vi "DMSO_EC_main_glass_cell_BM.vi"(0 "Constants":T5={"step to ml"=1920.0, "BoardNum"=1, "PosA BitNum"=6, "PosB BitNum"=5, "Heat Pulse Delay (ms)"=0.0, "Heating Iterations"=8, "N rinses"=2, "Dissolution Time (s)"=120, "SpargeBit"=0, "Extra Milli-Q (ml)"=2.0, "Valco Port Number"=6, "BitNum (Thermocouple)"=0, "Total Vol. (mL)"=12.0, "N syringe rinses"=2, "NaOH Vol (ml)"=2.0, "FanBit"=0}, 1 "Reduction Countdown Timer Refnum":refnum<vi>, 2 "Metadata":T1={"Local save location:"="C:\\Users\\bcamc\\OneDrive\\Desktop\\LabVIEW\\Test_metadata", "Cruise ID"="LaPerouse", "Sampling Timestamp"="2023-07-19 15:23:13", "Elution Timestamp"="2023-07-19 15:29:12", "GPS_Latitude"=-999.0, "GPS_Longitude"=-999.0, "DMS_std_conc"=0.0, "DMSP_std_conc"=0.0, "DMSO_std_conc"=0.0, "Std_index"=0.0, "Initial Trap Temp (oC)"=174.0, "Max Trap Temp (oC)"=174.0, "Final Trap Temp (oC)"=0.0, "Flow Rate (mL/min)"=0.0, "Comment"="", "GPS_Minute"=-999.0, "GPS_Day"=-999.0, "GPS_jd"=-999.0, "GPS_Hour"=-999.0, "GPS_Second"=-999.0, "GPS Baud"=4800.0, "COM Port (GPS)"="COM10", "Use GPS?"=FALSE, "Format Date"="%d-%d-%d"} {"GPS_Latitude" format="%_4g"; "GPS_Longitude" format="%_4g"; "GPS_jd" format="%_5g"; "Std_index" format="%.2g"; "DMSO_std_conc" format="%.2f"; "DMSP_std_conc" format="%.2f"; "DMS_std_conc" format="%.2f"}, 3 "Reduction Progress Bar Refnum":refnum<vi>, 4 "Sparging Countdown Timer Refnum":refnum<vi>, 5 "Sample Params":T4={"DMS Sparge Time (min)"=7.0, "Elution Time (min)"=1.5, "COM port (16 Pos. Valve)"="COM10", "Trap Heating Time (ms)"=675.0, "COM Port (DC Power)"="COM11", "COM Port (Runze)"="COM12", "sample volume"=10.0, "DMSO red. Sparge Time  (min)"=32.0, "DMSO Red. Duration (min)"=30.0, "Bypass sample handling (debugging)"=FALSE, "Reverse Reduction?"=FALSE, "Voltage (V)"="4.0", "DMSP Hydrolysis Time (min)"=13.0}, 6 "Sparging Progress Bar Refnum":refnum<vi>, 9 "Pump Parameters":T6={"Speed 1"="100", "Speed 2"="250", "Speed 3"="450", "Speed 4"="250", "UW/Sample"="5", "Sparge"="2", "Std"="4", "Waste"="15", "Air"="14", "Milli-Q"="1", "H2SO4"="6", "NaOH"="3", "Catalyst"="7", "Cell (H+ side)"="8", "Cell (sample side)"="9", "NaCl"="11"}, 10 "Elution Countdown Timer Refnum":refnum<vi>, 11 "Analysis Type":T3(ring)=enum."DMSO Only", 12 "Current Analyte Refnum":refnum<vi>, 14 "Temp Refnum":refnum<vi>, 15 "Elution Progress Bar Refnum":refnum<vi>) -> ()   [LabVIEW 2021]
uses:
  SubVIs/DMS-related/Sparge_stop.vi
  SubVIs/DMSO-related/Reduction_stop.vi
  SubVIs/DMS-related/Elution_stop.vi
  SubVIs/Refnum_control_global_BM.vi
  SubVIs/Plot_trap_heating_global_BM.vi
  SubVIs/DMSO-related/Temp_global_BM.vi
panel:
  out "Current Analyte":string
  in  "Mode Selection":T2(ring)
  out "Elution Progress Bar":u8(slide)=100 scale=0.0..100.0
  out "Sparging":bool
  out "Reduction Progress Bar":u8(slide)=100 scale=0.0..100.0
  out "Reduction Countdown (min)":dbl=-0.00026041666666666666 format="%.2g"
  out "Elution Countdown (min)":dbl=-0.0013020833333333333 format="%.2f"
  out "Error out":errorcluster
  out "Temp (oC)":i32=174
  in  "Error in":errorcluster
  out "Heating":bool
  out "Drying Flow":bool
  out "Sparge Countdown (min)":dbl=-0.00078125 format="%.2g"
  out "Sparging Progress Bar":u8(slide)=100 scale=0.0..100.0
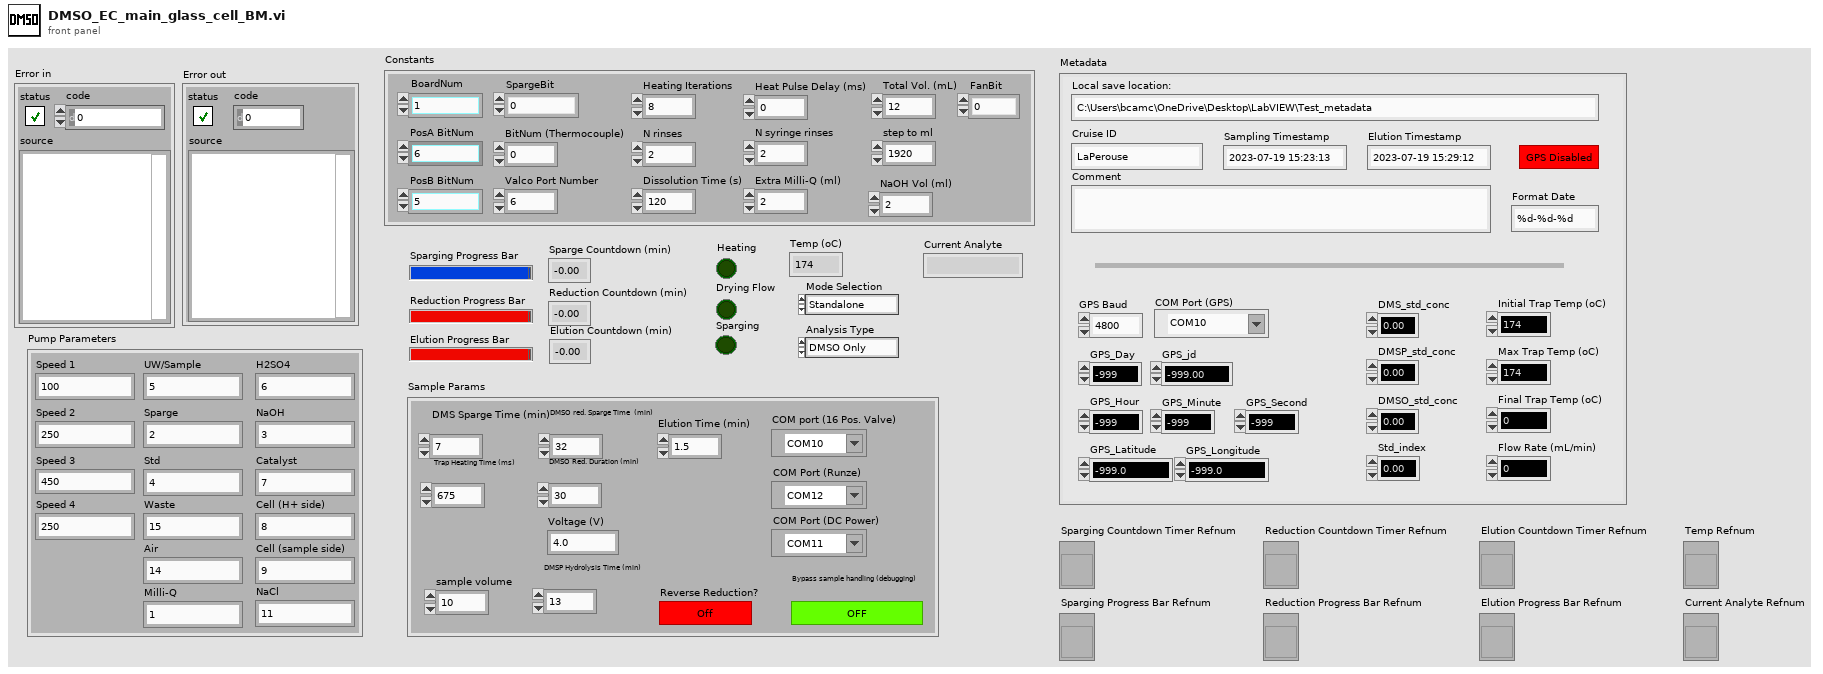
[diagram p1: front panel]
types:
  T1 = cluster{"Local save location:":string, "Cruise ID":string, "Sampling Timestamp":string, "Elution Timestamp":string, "GPS_Latitude":dbl, "GPS_Longitude":dbl, "DMS_std_conc":dbl, "DMSP_std_conc":dbl, "DMSO_std_conc":dbl, "Std_index":dbl, "Initial Trap Temp (oC)":dbl, "Max Trap Temp (oC)":dbl, "Final Trap Temp (oC)":dbl, "Flow Rate (mL/min)":dbl, "Comment":string, "GPS_Minute":dbl, "GPS_Day":dbl, "GPS_jd":dbl, "GPS_Hour":dbl, "GPS_Second":dbl, "GPS Baud":dbl, "COM Port (GPS)":refnum<visa-resource-name>, "Use GPS?":bool, "Format Date":string}
  T2 = enum16{"Standalone", "Standard Curve", "Point Std", "Analysis"}
  T3 = enum16{"DMS Only", "DMS/O", "DMS/P", "DMS/O/P", "DMSO Only"}
  T4 = cluster{"DMS Sparge Time (min)":dbl, "Elution Time (min)":dbl, "COM port (16 Pos. Valve)":refnum<visa-resource-name>, "Trap Heating Time (ms)":dbl, "COM Port (DC Power)":refnum<visa-resource-name>, "COM Port (Runze)":refnum<visa-resource-name>, "sample volume":dbl, "DMSO red. Sparge Time  (min)":dbl, "DMSO Red. Duration (min)":dbl, "Bypass sample handling (debugging)":bool, "Reverse Reduction?":bool, "Voltage (V)":string, "DMSP Hydrolysis Time (min)":dbl}
  T5 = cluster{"step to ml":dbl, "BoardNum":u32, "PosA BitNum":u32, "PosB BitNum":u32, "Heat Pulse Delay (ms)":dbl, "Heating Iterations":i32, "N rinses":i32, "Dissolution Time (s)":u32, "SpargeBit":u32, "Extra Milli-Q (ml)":dbl, "Valco Port Number":i32, "BitNum (Thermocouple)":u32, "Total Vol. (mL)":dbl, "N syringe rinses":i32, "NaOH Vol (ml)":dbl, "FanBit":u32}
  T6 = cluster{"Speed 1":string, "Speed 2":string, "Speed 3":string, "Speed 4":string, "UW/Sample":string, "Sparge":string, "Std":string, "Waste":string, "Air":string, "Milli-Q":string, "H2SO4":string, "NaOH":string, "Catalyst":string, "Cell (H+ side)":string, "Cell (sample side)":string, "NaCl":string}
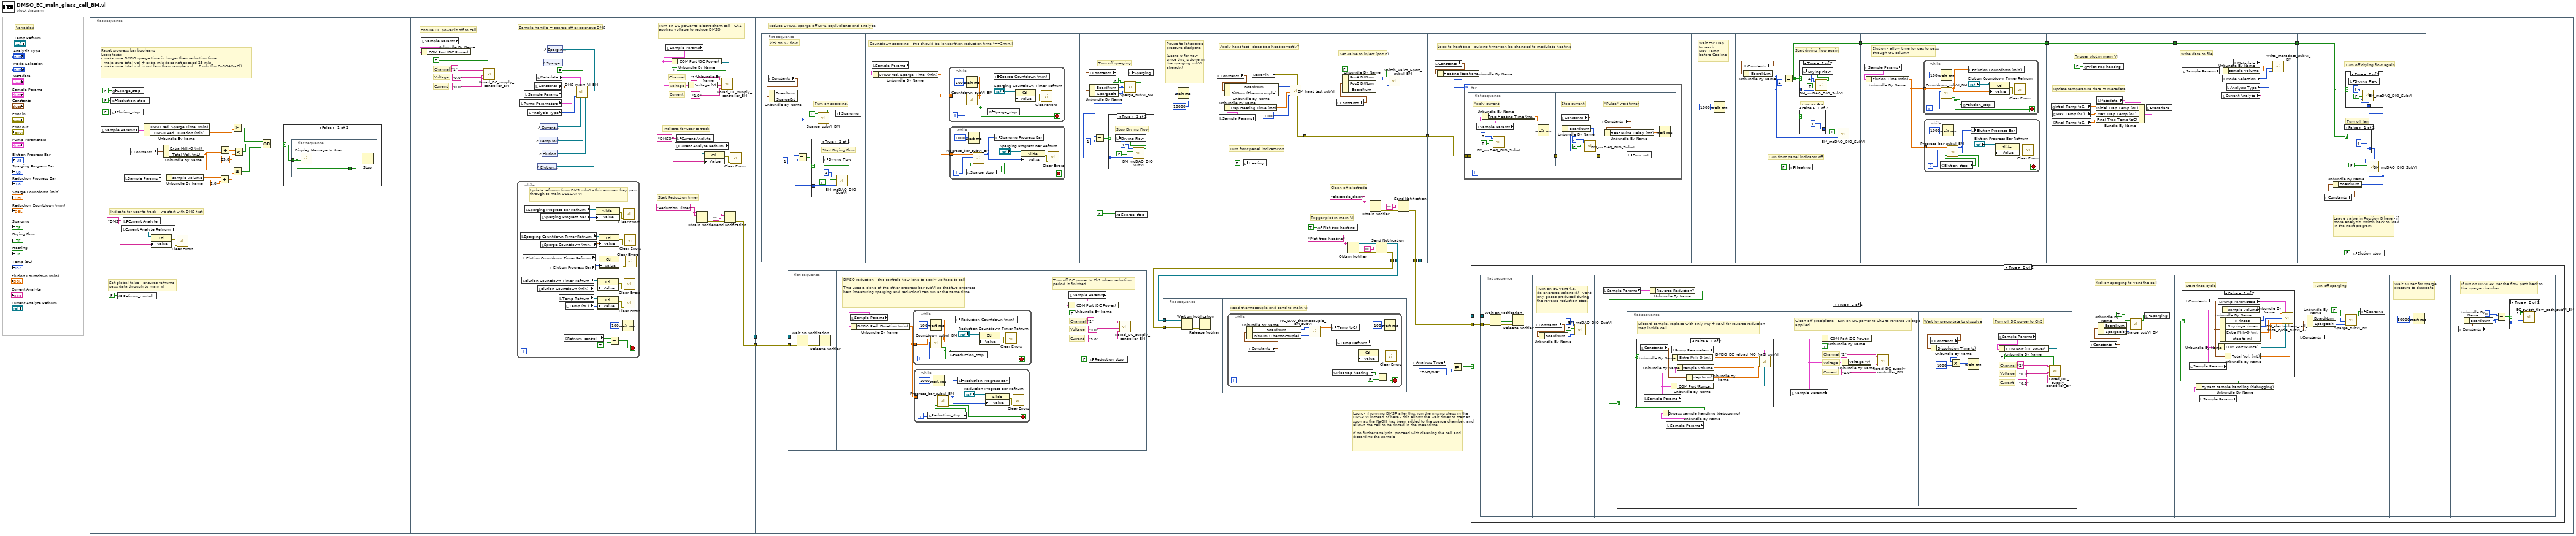
[diagram p0: block diagram]
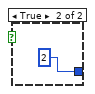
[diagram p10: hidden frame]
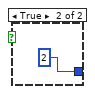
[diagram p12: hidden frame]
diagram:
  # "Variables"
  n1 = flat-sequence {
    tunnel: [w76] -> w2
    tunnel: [w75] -> w1
    tunnel: w2 -> [w93]
    tunnel: w1 -> [w92]
    frame #0 {
      w5 = "DMS" ("Current Analysis")
      # "Set global false - ensures refnums pass data through to main VI"
      # "Indicate for user to track -  we start with DMS first"
      # "Reset progress bar booleans\nLogic tests: \n- make sure DMSO sparge time is longer then reduction time\n- make sure total vol + extra mls does not exceed 25 mls\n- make sure total vol is not less than sample vol + 2 mls (for CuSO4/NaCl)"
      n2 = local read "Sample Params"() -> (w11:T4)
      n3 = global write "Reduction_stop.vi" "Reduction_stop"(FALSE ("Reduction_stop")) -> ()
      n4 = global write "Elution_stop.vi" "Elution_stop"(FALSE ("Elution_stop")) -> ()
      n5 = global write "Sparge_stop.vi" "Sparge_stop"(FALSE ("Stop_Reached")) -> ()
      n6 = global write "Refnum_control_global_BM.vi" "Refnum_control"(FALSE ("Refnum_control")) -> ()
      n7 = local read "Current Analyte Refnum"() -> (w6:refnum<vi>)
      n8 = local write "Current Analyte"(w5) -> ()
      n9 = local read "Sample Params"() -> (w8:T4)
      n10 = local read "Constants"() -> (w14:T5)
      n11 = Unbundle By Name(w11) -> ("DMSO red. Sparge Time  (min)"=w10:dbl, "DMSO Red. Duration (min)"=w9:dbl)
      n12 = property class="Ctl"(reference=w6, "Value"=w5) -> (error out=w4:errorcluster)  [unwired: 1 in, 1 out]
      n13 = Unbundle By Name(w14) -> ("Extra Milli-Q (ml)"=w13:dbl, "Total Vol. (mL)"=w12:dbl)
      n14 = Unbundle By Name(w8) -> ("sample volume"=w7:dbl)
      n15 = call <vilib>:"Clear Errors.vi"("error in (no error)"=w4) -> ()  [unwired: 5 in, 2 out]
      n16 = Add(x=w7, y=2.0) -> (x+y=w19:dbl)
      n17 = Add(x=w13, y=w12) -> (x+y=w22:dbl)
      n18 = Greater Or Equal?(x=w10, y=w9) -> (x >= y?=w18:bool)
      n19 = Greater Or Equal?(x=w12, y=w19) -> (x >= y?=w16:bool)
      n20 = Less?(x=w22, y=25.0) -> (x < y?=w17:bool)
      n21 = Compound Arithmetic op=OR(w18, w17, w16) -> (w15:bool)
      n22 = case shown="False" w15 {
        selector: w15 -> [w27 _]
        frame False {
          n23 = flat-sequence {
            tunnel: w27 -> [w28]
            tunnel: [w28] -> w26
            tunnel: w26 -> [w29]
            frame #0 {
              n24 = call "Display Message to User"("Enable"=w28) -> ()  [unwired: 9 in, 2 out]
            }
            frame #1 {
              n25 = Stop(stop? (T)=w29) -> ()
            }
          }
        }
        frame True {
          # "Else: carry on, nothing to see here..."
        }
      }
    }
    frame #1 {
      # "Channel"
      # "Ensure DC power is off to cell"
      # "Current"
      # "Voltage"
      n26 = local read "Sample Params"() -> (w31:T4)
      n27 = Unbundle By Name(w31) -> ("COM Port (DC Power)"=w30:refnum<visa-resource-name>)
      n28 = call "Korad_DC_supply_controller_BM.vi"("COM Port"=w30, "Master Output Control"=FALSE ("Output Control"), "Current"="0.0" ("Ch2 Current"), "Voltage"="0.0" ("Ch1 Voltage"), "Channel"="1" ("Ch1 Voltage")) -> ()  [unwired: 7 in]
    }
    frame #2 {
      # "Sample handle + sparge off exogenous DMS"
      n29 = while {
        stop <- w55 stop-if-true
        # "Update refnums from DMS subVI - this ensures they pass through to main OSSCAR VI"
        n30 = local read "Sparging Countdown Timer Refnum"() -> (w62:refnum<vi>)
        n31 = local read "Elution Countdown Timer Refnum"() -> (w50:refnum<vi>)
        n32 = local read "Elution Countdown Timer Refnum"() -> (w53:refnum<vi>)
        n33 = local read "Sparging Progress Bar Refnum"() -> (w65:refnum<vi>)
        n34 = local read "Elution Countdown (min)"() -> (w51:dbl)
        n35 = local read "Sparging Progress Bar"() -> (w64:u8)
        n36 = local read "Sparge Countdown (min)"() -> (w63:dbl)
        n37 = local read "Elution Progress Bar"() -> (w52:u8)
        n38 = local read "Temp Refnum"() -> (w59:refnum<vi>)
        n39 = global read "Refnum_control_global_BM.vi" "Refnum_control"() -> (w57:bool)
        n40 = local read "Temp (oC)"() -> (w58:i32)
        n41 = property class="Slide"(reference=w65, "Value"=w64) -> (error out=w66:errorcluster)  [unwired: 1 in, 1 out]
        n42 = property class="Ctl"(reference=w50, "Value"=w51) -> (error out=w49:errorcluster)  [unwired: 1 in, 1 out]
        n43 = property class="Ctl"(reference=w59, "Value"=w58) -> (error out=w60:errorcluster)  [unwired: 1 in, 1 out]
        n44 = property class="Ctl"(reference=w62, "Value"=w63) -> (error out=w61:errorcluster)  [unwired: 1 in, 1 out]
        n45 = property class="Ctl"(reference=w53, "Value"=w52) -> (error out=w54:errorcluster)  [unwired: 1 in, 1 out]
        n46 = Equal?(x=w57, y=TRUE) -> (x = y?=w55:bool)
        n47 = Wait (ms)(milliseconds to wait=u32 100) -> ()  [unwired: 1 out]
        n48 = call <vilib>:"Clear Errors.vi"("error in (no error)"=w66) -> ()  [unwired: 5 in, 2 out]
        n49 = call <vilib>:"Clear Errors.vi"("error in (no error)"=w49) -> ()  [unwired: 5 in, 2 out]
        n50 = call <vilib>:"Clear Errors.vi"("error in (no error)"=w60) -> ()  [unwired: 5 in, 2 out]
        n51 = call <vilib>:"Clear Errors.vi"("error in (no error)"=w61) -> ()  [unwired: 5 in, 2 out]
        n52 = call <vilib>:"Clear Errors.vi"("error in (no error)"=w54) -> ()  [unwired: 5 in, 2 out]
      }
      n53 = local read "Pump Parameters"() -> (w45:T6)
      n54 = local read "Sample Params"() -> (w46:T4)
      n55 = local read "Analysis Type"() -> (w44:T3)
      n56 = local read "Constants"() -> (w47:T5)
      n57 = local read "Metadata"() -> (w43:T1)
      n58 = control-ref of="Elution Countdown (min)"() -> (w39:refnum<vi>)
      n59 = control-ref of="Temp (oC)"() -> (w38:refnum<vi>)
      n60 = control-ref of="Current Analyte"() -> (w37:refnum<vi>)
      n61 = control-ref of="Elution Progress Bar"() -> (w40:refnum<vi>)
      n62 = control-ref of="Sparge Countdown (min)"() -> (w41:refnum<vi>)
      n63 = control-ref of="Sparging Progress Bar"() -> (w36:refnum<vi>)
      n64 = call "DMS_main_VI_BM.vi"("Elution Progress Bar Refnum"=w40, "Elution Countdown Timer Refnum"=w39, "Sparging Progress Bar Refnum"=w36, "Sparging Countdown Timer Refnum"=w41, "Temp Refnum"=w38, "Skip sample handling"=FALSE, "Current Analyte Refnum"=w37, "Metadata"=w43, "Analysis Type"=w44, "Pump Parameters"=w45, "Sample Params"=w46, "Constants"=w47) -> ()
    }
    frame #3 {
      w68 = "DMSO" ("Current Analysis")
      w78 = "Reduction Timer"
      # "Indicate for user to track"
      # "Channel"
      # "Current"
      # "Voltage"
      # "Start Reduction timer"
      # "Turn on DC power to electrochem cell - Ch1 applies voltage to reduce DMSO"
      n65 = local read "Sample Params"() -> (w70:T4)
      n66 = Unbundle By Name(w70) -> ("COM Port (DC Power)"=w72:refnum<visa-resource-name>)
      n67 = local read "Current Analyte Refnum"() -> (w67:refnum<vi>)
      n68 = local write "Current Analyte"(w68) -> ()
      n69 = Unbundle By Name(w70) -> ("Voltage (V)"=w71:string)
      n70 = Obtain Notifier(name (unnamed)=w78, notification data type=w78) -> (notifier out=w80:refnum<notifier>, error out=w79:errorcluster)  [unwired: 2 in, 1 out]
      n71 = property class="Ctl"(reference=w67, "Value"=w68) -> (error out=w69:errorcluster)  [unwired: 1 in, 1 out]
      n72 = call "Korad_DC_supply_controller_BM.vi"("COM Port"=w72, "Master Output Control"=TRUE ("Output Control"), "Current"="1.0" ("Ch2 Current"), "Voltage"=w71, "Channel"="1" ("Ch1 Voltage")) -> ()  [unwired: 7 in]
      n73 = Send Notification(notification="", notifier=w80, error in (no error)=w79) -> (notifier out=w76:refnum<notifier>, error out=w75:errorcluster)
      n74 = call <vilib>:"Clear Errors.vi"("error in (no error)"=w69) -> ()  [unwired: 5 in, 2 out]
    }
    frame #4 {
      # "Logic - if running DMSP after this, run the rinsing steps in the DMSP VI instead of here - this allows the wait timer to start as soon as the NaOH has been added to the sparge chamber, and allows the cell to be rinsed in the meantime\n\nIf no further analysis, proceed with cleaning the cell and discarding the sample"
      # "Reduce DMSO, sparge off DMS equivalents and analyze"
      n75 = flat-sequence {
        tunnel: [w254] -> w96
        tunnel: [w274] -> w95
        tunnel: w96 -> [w274]
        tunnel: [w269] -> w91
        tunnel: [w268] -> w90
        tunnel: [w258] -> w82
        tunnel: [w257] -> w83
        tunnel: w95 -> [w278]
        tunnel: [w301] -> w94
        tunnel: [w311] -> w85
        tunnel: w94 -> [w311]
        tunnel: w85 -> [w333]
        tunnel: [w333] -> w84
        tunnel: w84 -> [w340]
        tunnel: [w340] -> w86
        tunnel: w86 -> [w344]
        frame #0 {
          # "Turn on sparging."
          # "kick on N2 flow"
          n76 = local read "Constants"() -> (w209:T5)
          n77 = Unbundle By Name(w209) -> ("BoardNum"=w208:u32, "SpargeBit"=w207:u32)
          n78 = Equal?(x=w208, y=u32 1) -> (x = y?=w213:bool)
          n79 = case shown="True" w213 {
            tunnel: w208 -> [_ w214]
            frame False {
            }
            frame True {
              # "Start Drying Flow"
              n80 = call "BM_mcDAQ_DIO_SubVI.vi"("BoardNum"=w214, "BitValue"=TRUE, "BitNum"=4) -> ("Control out"=w217:bool)  [unwired: 8 in]
              n81 = local write "Drying Flow"(w217) -> ()
            }
          }
          n82 = call "Sparge_subVI_BM.vi"("BitNum"=w207, "BoardNum"=w208, "Sparge now"=TRUE) -> ("Sparging"=w210:bool)  [unwired: 8 in]
          n83 = local write "Sparging"(w210) -> ()
        }
        frame #1 {
          # "Countdown sparging - this should be longer than reduction time (~+2min)!"
          n84 = local read "Sample Params"() -> (w219:T4)
          n85 = Unbundle By Name(w219) -> ("DMSO red. Sparge Time  (min)"=w218:dbl)
          n86 = while {
            tunnel: w218 -> [w229]
            i -> [w233]
            stop <- w232 stop-if-true
            n87 = Wait (ms)(milliseconds to wait=u32 100) -> ()  [unwired: 1 out]
            n88 = call "Countdown_subVI_BM.vi"("Current Iteration"=w233, "Runtime (min)"=w229) -> ("Global Stop"=w232:bool, "Countdown Timer (min)"=w230:dbl)  [unwired: 8 in]
            n89 = global write "Sparge_stop.vi" "Sparge_stop"(w232) -> ()
            n90 = local write "Sparge Countdown (min)"(w230) -> ()
            n91 = property class="Ctl"(reference="Sparging Countdown Timer Refnum", "Value"=w230) -> (error out=w228:errorcluster)  [unwired: 1 in, 1 out]
            n92 = call <vilib>:"Clear Errors.vi"("error in (no error)"=w228) -> ()  [unwired: 5 in, 2 out]
          }
          n93 = while {
            tunnel: w218 -> [w221]
            i -> [w226]
            stop <- w224 stop-if-true
            n94 = global read "Sparge_stop.vi" "Sparge_stop"() -> (w225:bool)
            n95 = Wait (ms)(milliseconds to wait=u32 1000) -> ()  [unwired: 1 out]
            n96 = call "Progress_bar_subVI_BM.vi"("Global Stop"=w225, "Current Iteration"=w226, "Runtime (min)"=w221) -> ("Loop Stop"=w224:bool, "Progress Bar"=w222:u8)  [unwired: 7 in]
            n97 = local write "Sparging Progress Bar"(w222) -> ()
            n98 = property class="Slide"(reference="Sparging Progress Bar Refnum", "Value"=w222) -> (error out=w220:errorcluster)  [unwired: 1 in, 1 out]
            n99 = call <vilib>:"Clear Errors.vi"("error in (no error)"=w220) -> ()  [unwired: 5 in, 2 out]
          }
        }
        frame #2 {
          # "Turn off sparging"
          n100 = local read "Constants"() -> (w237:T5)
          n101 = Unbundle By Name(w237) -> ("BoardNum"=w235:u32, "SpargeBit"=w236:u32)
          n102 = Equal?(x=w235, y=u32 1) -> (x = y?=w242:bool)
          n103 = case shown="True" w242 {
            tunnel: w235 -> [_ w244]
            frame False {
            }
            frame True {
              # "Stop Drying Flow"
              n104 = call "BM_mcDAQ_DIO_SubVI.vi"("BoardNum"=w244, "BitValue"=FALSE, "BitNum"=4) -> ("Control out"=w243:bool)  [unwired: 8 in]
              n105 = local write "Drying Flow"(w243) -> ()
            }
          }
          n106 = global write "Sparge_stop.vi" "Sparge_stop"(FALSE ("Stop_Reached")) -> ()
          n107 = call "Sparge_subVI_BM.vi"("BitNum"=w236, "BoardNum"=w235, "Sparge now"=FALSE) -> ("Sparging"=w239:bool)  [unwired: 8 in]
          n108 = local write "Sparging"(w239) -> ()
        }
        frame #3 {
          # "Pause to let sparge\npressure dissipate\n\n(Set to 0 for now since this is done in the sparging subVI already)"
          n109 = Wait (ms)(milliseconds to wait=10000) -> ()  [unwired: 1 out]
        }
        frame #4 {
          # "Turn front panel indicator on"
          # "Apply heat test - does trap heat correctly?"
          n110 = local read "Constants"() -> (w252:T5)
          n111 = local read "Sample Params"() -> (w250:T4)
          n112 = Unbundle By Name(w252) -> ("BoardNum"=w251:u32, "BitNum (Thermocouple)"=w248:u32)
          n113 = Unbundle By Name(w250) -> ("Trap Heating Time (ms)"=w249:dbl)
          n114 = local write "Heating"(TRUE ("Heating")) -> ()
          n115 = local read "Error in"() -> (w256:errorcluster)
          n116 = call "BM_heat_test_subVI.vi"("error in (no error)"=w256, "Heat Pulse Delay (ms)"=u32 1000, "Trap Heating Time (ms)"=w249, "BitNum"=w248, "BoardNum"=w251) -> ("error out"=w254:errorcluster)  [unwired: 6 out]
        }
        frame #5 {
          w260 = "Plot_trap_heating"
          w272 = "Electrode_clean"
          # "Trigger plot in main VI"
          # "Clean off electrode"
          # "Set valve to inject (pos B)"
          n117 = global write "Plot_trap_heating_global_BM.vi" "Plot trap heating"(TRUE ("Plot trap heating")) -> ()
          n118 = local read "Constants"() -> (w267:T5)
          n119 = Unbundle By Name(w267) -> ("PosA BitNum"=w266:u32, "PosB BitNum"=w265:u32, "BoardNum"=w264:u32)
          n120 = Obtain Notifier(name (unnamed)=w260, notification data type=w260) -> (notifier out=w263:refnum<notifier>, error out=w262:errorcluster)  [unwired: 2 in, 1 out]
          n121 = Obtain Notifier(name (unnamed)=w272, notification data type=w272) -> (notifier out=w271:refnum<notifier>, error out=w270:errorcluster)  [unwired: 2 in, 1 out]
          n122 = Send Notification(notification="", notifier=w263, error in (no error)=w262) -> (notifier out=w258:refnum<notifier>, error out=w257:errorcluster)
          n123 = call "Switch_Valco_6port_subVI_BM.vi"("Load (T) or Inject (F)"=FALSE, "PosA BitNum"=w266, "PosB BitNum"=w265, "BoardNum"=w264) -> ()  [unwired: 6 in, 1 out]
          n124 = Send Notification(notification="", notifier=w271, error in (no error)=w270) -> (notifier out=w269:refnum<notifier>, error out=w268:errorcluster)
        }
        frame #6 {
          # "Loop to heat trap - pulsing timer can be changed to modulate heating"
          n125 = local read "Constants"() -> (w277:T5)
          n126 = Unbundle By Name(w277) -> ("Heating Iterations"=w276:i32)
          n127 = for {
            N: w276 -> [_]
            tunnel: w278 -> [w281]
            n128 = flat-sequence {
              tunnel: [w284] -> w279
              tunnel: w281 -> [w284]
              tunnel: [w289] -> w280
              tunnel: w279 -> [w289]
              tunnel: w280 -> [w292]
              frame #0 {
                # "Apply current"
                n129 = local read "Sample Params"() -> (w282:T4)
                n130 = Unbundle By Name(w282) -> ("Trap Heating Time (ms)"=w283:dbl)
                n131 = call "BM_mcDAQ_DIO_SubVI.vi"("BitValue"=TRUE, "BitNum"=7) -> ()  [unwired: 9 in, 1 out]
                n132 = Wait (ms)(milliseconds to wait=w283) -> ()  [unwired: 1 out]
              }
              frame #1 {
                # "Stop current"
                n133 = local read "Constants"() -> (w288:T5)
                n134 = Unbundle By Name(w288) -> ("BoardNum"=w287:u32)
                n135 = call "BM_mcDAQ_DIO_SubVI.vi"("BoardNum"=w287, "BitValue"=FALSE, "BitNum"=7) -> ()  [unwired: 8 in, 1 out]
              }
              frame #2 {
                # "\"Pulse\" wait timer"
                n136 = local read "Constants"() -> (w294:T5)
                n137 = Unbundle By Name(w294) -> ("Heat Pulse Delay (ms)"=w293:dbl)
                n138 = local write "Error out"(w292) -> ()
                n139 = Wait (ms)(milliseconds to wait=w293) -> ()  [unwired: 1 out]
              }
            }
          }
        }
        frame #7 {
          # "Wait For Trap\nto reach\nMax Temp \nbefore Cooling"
          n140 = Wait (ms)(milliseconds to wait=1000) -> ()  [unwired: 1 out]
        }
        frame #8 {
          # "Turn on fan"
          # "Turn front panel indicator off"
          # "Start drying flow again"
          n141 = local read "Constants"() -> (w296:T5)
          n142 = Unbundle By Name(w296) -> ("BoardNum"=w297:u32)
          n143 = Equal?(x=w297, y=u32 1) -> (x = y?=w301:bool)
          n144 = local write "Heating"(FALSE ("Heating")) -> ()
          n145 = case shown="True" w301 {
            tunnel: w297 -> [_ w305]
            frame False {
            }
            frame True {
              n146 = call "BM_mcDAQ_DIO_SubVI.vi"("BoardNum"=w305, "BitValue"=TRUE, "BitNum"=u32 4) -> ("Control out"=w306:bool)  [unwired: 8 in]
              n147 = local write "Drying Flow"(w306) -> ()
            }
          }
          n148 = case shown="False" w301 {
            tunnel: [u32 4 ("BitNum") u32 2 ("BitNum")] -> w299
            frame False {
            }
            frame True {
            }
          }
          n149 = call "BM_mcDAQ_DIO_SubVI.vi"("BoardNum"=w297, "BitValue"=TRUE, "BitNum"=w299) -> ()  [unwired: 8 in, 1 out]
        }
        frame #9 {
          # "Elution - allow time for gas to pass through GC column"
          n150 = local read "Sample Params"() -> (w310:T4)
          n151 = Unbundle By Name(w310) -> ("Elution Time (min)"=w309:dbl)
          n152 = while {
            tunnel: w309 -> [w321]
            i -> [w325]
            stop <- w324 stop-if-true
            n153 = Wait (ms)(milliseconds to wait=u32 100) -> ()  [unwired: 1 out]
            n154 = call "Countdown_subVI_BM.vi"("Current Iteration"=w325, "Runtime (min)"=w321) -> ("Global Stop"=w324:bool, "Countdown Timer (min)"=w322:dbl)  [unwired: 8 in]
            n155 = global write "Elution_stop.vi" "Elution_stop"(w324) -> ()
            n156 = local write "Elution Countdown (min)"(w322) -> ()
            n157 = property class="Ctl"(reference="Elution Countdown Timer Refnum", "Value"=w322) -> (error out=w320:errorcluster)  [unwired: 1 in, 1 out]
            n158 = call <vilib>:"Clear Errors.vi"("error in (no error)"=w320) -> ()  [unwired: 5 in, 2 out]
          }
          n159 = while {
            tunnel: w309 -> [w313]
            i -> [w318]
            stop <- w316 stop-if-true
            n160 = global read "Elution_stop.vi" "Elution_stop"() -> (w317:bool)
            n161 = Wait (ms)(milliseconds to wait=u32 1000) -> ()  [unwired: 1 out]
            n162 = call "Progress_bar_subVI_BM.vi"("Global Stop"=w317, "Current Iteration"=w318, "Runtime (min)"=w313) -> ("Loop Stop"=w316:bool, "Progress Bar"=w314:u8)  [unwired: 7 in]
            n163 = local write "Elution Progress Bar"(w314) -> ()
            n164 = property class="Slide"(reference="Elution Progress Bar Refnum", "Value"=w314) -> (error out=w312:errorcluster)  [unwired: 1 in, 1 out]
            n165 = call <vilib>:"Clear Errors.vi"("error in (no error)"=w312) -> ()  [unwired: 5 in, 2 out]
          }
        }
        frame #10 {
          # "Update temperature data to metadata"
          # "Trigger plot in main VI"
          n166 = global read "Temp_global_BM.vi" "Intial Temp (oC)"() -> (w329:dbl)
          n167 = global read "Temp_global_BM.vi" "Final Temp (oC)"() -> (w331:dbl)
          n168 = global read "Temp_global_BM.vi" "Max Temp (oC)"() -> (w330:dbl)
          n169 = global write "Plot_trap_heating_global_BM.vi" "Plot trap heating"(FALSE ("Plot trap heating")) -> ()
          n170 = local read "Metadata"() -> (w327:T1)
          n171 = Bundle By Name(cluster=w327, "Initial Trap Temp (oC)"=w329, "Max Trap Temp (oC)"=w330, "Final Trap Temp (oC)"=w331) -> (w328:T1)
          n172 = local write "Metadata"(w328) -> ()
        }
        frame #11 {
          # "Write data to file"
          n173 = local read "Sample Params"() -> (w339:T4)
          n174 = local read "Current Analyte"() -> (w334:string)
          n175 = local read "Mode Selection"() -> (w336:T2)
          n176 = Unbundle By Name(w339) -> ("sample volume"=w337:dbl)
          n177 = local read "Analysis Type"() -> (w335:T3)
          n178 = local read "Metadata"() -> (w338:T1)
          n179 = call "Write_metadata_subVI_BM.vi"("Analyte"=w334, "Analysis Type"=w335, "Mode Selection"=w336, "sample volume"=w337, "Metadata"=w338) -> ()  [unwired: 7 in]
        }
        frame #12 {
          # "Leave valve in Position B here - if more analysis, switch back to load in the next program"
          # "Turn off fan"
          # "Turn off drying flow again"
          n180 = local read "Constants"() -> (w342:T5)
          n181 = Unbundle By Name(w342) -> ("BoardNum"=w341:u32)
          n182 = case shown="False" w344 {
            tunnel: [u32 4 ("BitNum") u32 2 ("BitNum")] -> w346
            frame False {
            }
            frame True {
            }
          }
          n183 = case shown="True" w344 {
            tunnel: w341 -> [_ w350]
            frame False {
            }
            frame True {
              n184 = call "BM_mcDAQ_DIO_SubVI.vi"("BoardNum"=w350, "BitValue"=FALSE, "BitNum"=u32 4) -> ("Control out"=w349:bool)  [unwired: 8 in]
              n185 = local write "Drying Flow"(w349) -> ()
            }
          }
          n186 = global write "Elution_stop.vi" "Elution_stop"(FALSE ("Elution_stop")) -> ()
          n187 = call "BM_mcDAQ_DIO_SubVI.vi"("BoardNum"=w341, "BitValue"=FALSE, "BitNum"=w346) -> ()  [unwired: 8 in, 1 out]
        }
      }
      n188 = flat-sequence {
        tunnel: w93 -> [w179]
        tunnel: w92 -> [w178]
        frame #0 {
          n189 = Wait on Notification(notifier=w179, error in (no error)=w178) -> (notifier out=w182:refnum<notifier>, timed out?=w181:bool, error out=w180:errorcluster)  [unwired: 3 out]
          n190 = Release Notifier(notifier=w182, force destroy? (F)=w181, error in (no error)=w180) -> ()  [unwired: 3 out]
        }
        frame #1 {
          # "DMSO reduction - this controls how long to apply voltage to cell\n\nThis uses a clone of the other progress bar subVI so that two progress bars (measuring sparging and reduction) can run at the same time."
          n191 = local read "Sample Params"() -> (w184:T4)
          n192 = Unbundle By Name(w184) -> ("DMSO Red. Duration (min)"=w183:dbl)
          n193 = while {
            tunnel: w183 -> [w198]
            i -> [w197]
            stop <- w196 stop-if-true
            n194 = Wait (ms)(milliseconds to wait=u32 100) -> ()  [unwired: 1 out]
            n195 = call "Countdown_subVI_BM.vi"("Current Iteration"=w197, "Runtime (min)"=w198) -> ("Global Stop"=w196:bool, "Countdown Timer (min)"=w194:dbl)  [unwired: 8 in]
            n196 = global write "Reduction_stop.vi" "Reduction_stop"(w196) -> ()
            n197 = local write "Reduction Countdown (min)"(w194) -> ()
            n198 = property class="Ctl"(reference="Reduction Countdown Timer Refnum", "Value"=w194) -> (error out=w193:errorcluster)  [unwired: 1 in, 1 out]
            n199 = call <vilib>:"Clear Errors.vi"("error in (no error)"=w193) -> ()  [unwired: 5 in, 2 out]
          }
          n200 = while {
            tunnel: w183 -> [w191]
            i -> [w190]
            stop <- w188 stop-if-true
            n201 = global read "Reduction_stop.vi" "Reduction_stop"() -> (w189:bool)
            n202 = Wait (ms)(milliseconds to wait=u32 1000) -> ()  [unwired: 1 out]
            n203 = call "Progress_bar_subVI_BM.vi"("Global Stop"=w189, "Current Iteration"=w190, "Runtime (min)"=w191) -> ("Loop Stop"=w188:bool, "Progress Bar"=w186:u8)  [unwired: 7 in]
            n204 = local write "Reduction Progress Bar"(w186) -> ()
            n205 = property class="Slide"(reference="Reduction Progress Bar Refnum", "Value"=w186) -> (error out=w185:errorcluster)  [unwired: 1 in, 1 out]
            n206 = call <vilib>:"Clear Errors.vi"("error in (no error)"=w185) -> ()  [unwired: 5 in, 2 out]
          }
        }
        frame #2 {
          # "Channel"
          # "Current"
          # "Voltage"
          # "Turn off DC power to Ch1 when reduction period is finished"
          n207 = local read "Sample Params"() -> (w201:T4)
          n208 = Unbundle By Name(w201) -> ("COM Port (DC Power)"=w200:refnum<visa-resource-name>)
          n209 = global write "Reduction_stop.vi" "Reduction_stop"(FALSE ("Reduction_stop")) -> ()
          n210 = call "Korad_DC_supply_controller_BM.vi"("COM Port"=w200, "Master Output Control"=FALSE ("Output Control"), "Current"="0.0" ("Ch2 Current"), "Voltage"="0.0" ("Ch1 Voltage"), "Channel"="1" ("Ch1 Voltage")) -> ()  [unwired: 7 in]
        }
      }
      n211 = flat-sequence {
        tunnel: w82 -> [w98]
        tunnel: w83 -> [w97]
        frame #0 {
          n212 = Wait on Notification(notifier=w98, error in (no error)=w97) -> (notifier out=w100:refnum<notifier>, error out=w99:errorcluster)  [unwired: 4 out]
          n213 = Release Notifier(notifier=w100, error in (no error)=w99) -> ()  [unwired: 1 in, 3 out]
        }
        frame #1 {
          # "Read thermocouple and send to main VI"
          n214 = while {
            stop <- w103 stop-if-true
            n215 = local read "Constants"() -> (w108:T5)
            n216 = Unbundle By Name(w108) -> ("BoardNum"=w109:u32, "BitNum (Thermocouple)"=w110:u32)
            n217 = call "MC_DAQ_thermocouple_BM_subVI.vi"("BitNum"=w110, "BoardNum"=w109) -> ("Temp (oC)"=w107:dbl)  [unwired: 8 in, 1 out]
            n218 = local write "Temp (oC)"(w107) -> ()
            n219 = global read "Plot_trap_heating_global_BM.vi" "Plot trap heating"() -> (w104:bool)
            n220 = local read "Temp Refnum"() -> (w106:refnum<vi>)
            n221 = property class="Ctl"(reference=w106, "Value"=w107) -> (error out=w105:errorcluster)  [unwired: 1 in, 1 out]
            n222 = Equal?(x=w104, y=FALSE) -> (x = y?=w103:bool)
            n223 = Wait (ms)(milliseconds to wait=u32 100) -> ()  [unwired: 1 out]
            n224 = call <vilib>:"Clear Errors.vi"("error in (no error)"=w105) -> ()  [unwired: 5 in, 2 out]
          }
        }
      }
      n225 = local read "Analysis Type"() -> (w88:T3)
      n226 = Not Equal?(x=w88, y=T3."DMS/O/P" ("x")) -> (x != y?=w87:bool)
      n227 = case shown="True" w87 {
        tunnel: w91 -> [_ w112]
        tunnel: w90 -> [_ w111]
        frame False {
        }
        frame True {
          n228 = flat-sequence {
            tunnel: w112 -> [w114]
            tunnel: w111 -> [w113]
            frame #0 {
              n229 = Wait on Notification(notifier=w114, error in (no error)=w113) -> (notifier out=w115:refnum<notifier>, timed out?=w117:bool, error out=w116:errorcluster)  [unwired: 3 out]
              n230 = Release Notifier(notifier=w115, force destroy? (F)=w117, error in (no error)=w116) -> ()  [unwired: 3 out]
            }
            frame #1 {
              # "Turn on EC vent (i.e. de-energize solenoid) - vent any gases produced during the reverse reduction step."
              n231 = local read "Constants"() -> (w121:T5)
              n232 = Unbundle By Name(w121) -> ("BoardNum"=w120:u32)
              n233 = call "BM_mcDAQ_DIO_SubVI.vi"("BoardNum"=w120, "BitValue"=FALSE, "BitNum"=u32 3) -> ()  [unwired: 8 in, 1 out]
            }
            frame #2 {
              n234 = local read "Sample Params"() -> (w123:T4)
              n235 = Unbundle By Name(w123) -> ("Reverse Reduction?"=w122:bool)
              n236 = case shown="True" w122 {
                frame False {
                  # "Skip to rinsing out the cell"
                }
                frame True {
                  n237 = flat-sequence {
                    frame #0 {
                      # "Discard sample, replace with only MQ + NaCl for reverse reduction step inside cell"
                      n238 = local read "Sample Params"() -> (w125:T4)
                      n239 = Unbundle By Name(w125) -> ("Bypass sample handling (debugging)"=w124:bool)
                      n240 = case shown="False" w124 {
                        frame False {
                          n241 = local read "Constants"() -> (w129:T5)
                          n242 = local read "Sample Params"() -> (w126:T4)
                          n243 = Unbundle By Name(w126) -> ("COM Port (Runze)"=w127:refnum<visa-resource-name>)
                          n244 = local read "Pump Parameters"() -> (w132:T6)
                          n245 = Unbundle By Name(w129) -> ("Extra Milli-Q (ml)"=w131:dbl)
                          n246 = Unbundle By Name(w126) -> ("sample volume"=w128:dbl)
                          n247 = Unbundle By Name(w129) -> ("step to ml"=w130:dbl)
                          n248 = call "DMSO_EC_reload_MQ_NaCl_subVI.vi"("COM Port"=w127, "Pump Parameters"=w132, "step to ml"=w130, "Sample Vol. (mL)"=w128, "Extra Milli-Q (ml)"=w131) -> ()  [unwired: 7 in]
                        }
                        frame True {
                        }
                      }
                    }
                    frame #1 {
                      # "Channel"
                      # "Current"
                      # "Voltage"
                      # "Clean off precipitate - turn on DC power to Ch2 to reverse voltage applied"
                      n249 = local read "Sample Params"() -> (w133:T4)
                      n250 = Unbundle By Name(w133) -> ("COM Port (DC Power)"=w135:refnum<visa-resource-name>)
                      n251 = Unbundle By Name(w133) -> ("Voltage (V)"=w134:string)
                      n252 = call "Korad_DC_supply_controller_BM.vi"("COM Port"=w135, "Master Output Control"=TRUE ("Output Control"), "Current"="1.0" ("Ch2 Current"), "Voltage"=w134, "Channel"="2" ("Ch1 Voltage")) -> ()  [unwired: 7 in]
                    }
                    frame #2 {
                      # "Wait for precipitate to dissolve"
                      n253 = local read "Constants"() -> (w140:T5)
                      n254 = Unbundle By Name(w140) -> ("Dissolution Time (s)"=w139:u32)
                      n255 = Multiply(x=w139, y=u32 1000) -> (x*y=w142:u32)
                      n256 = Wait (ms)(milliseconds to wait=w142) -> ()  [unwired: 1 out]
                    }
                    frame #3 {
                      # "Channel"
                      # "Current"
                      # "Voltage"
                      # "Turn off DC power to Ch2"
                      n257 = local read "Sample Params"() -> (w144:T4)
                      n258 = Unbundle By Name(w144) -> ("COM Port (DC Power)"=w143:refnum<visa-resource-name>)
                      n259 = call "Korad_DC_supply_controller_BM.vi"("COM Port"=w143, "Master Output Control"=FALSE ("Output Control"), "Current"="0.0" ("Ch2 Current"), "Voltage"="0.0" ("Ch1 Voltage"), "Channel"="2" ("Ch1 Voltage")) -> ()  [unwired: 7 in]
                    }
                  }
                }
              }
            }
            frame #3 {
              # "Kick on sparging to vent the cell"
              n260 = local read "Constants"() -> (w151:T5)
              n261 = Unbundle By Name(w151) -> ("BoardNum"=w150:u32, "SpargeBit"=w149:u32)
              n262 = call "Sparge_subVI_BM.vi"("BitNum"=w149, "BoardNum"=w150, "Sparge now"=TRUE) -> ("Sparging"=w152:bool)  [unwired: 8 in]
              n263 = local write "Sparging"(w152) -> ()
            }
            frame #4 {
              # "Start rinse cycle"
              n264 = local read "Sample Params"() -> (w154:T4)
              n265 = Unbundle By Name(w154) -> ("Bypass sample handling (debugging)"=w155:bool)
              n266 = case shown="False" w155 {
                frame False {
                  n267 = local read "Constants"() -> (w161:T5)
                  n268 = local read "Sample Params"() -> (w158:T4)
                  n269 = local read "Pump Parameters"() -> (w165:T6)
                  n270 = Unbundle By Name(w158) -> ("COM Port (Runze)"=w159:refnum<visa-resource-name>)
                  n271 = Unbundle By Name(w161) -> ("N rinses"=w157:i32, "N syringe rinses"=w156:i32, "Extra Milli-Q (ml)"=w164:dbl, "step to ml"=w163:dbl)
                  n272 = Unbundle By Name(w158) -> ("sample volume"=w160:dbl)
                  n273 = Unbundle By Name(w161) -> ("Total Vol. (mL)"=w162:dbl)
                  n274 = call "BM_electrochem_cell_rinse_cycle_subVI_v2.vi"("Sample Volume"=w160, "Pump Parameters"=w165, "N cell rinses"=w157, "N syringe rinses"=w156, "Extra Milli-Q (ml)"=w164, "step to ml"=w163, "COM Port"=w159, "Total Vol. (mL)"=w162) -> ()  [unwired: 8 in]
                }
                frame True {
                }
              }
            }
            frame #5 {
              # "Turn off sparging"
              n275 = local read "Constants"() -> (w168:T5)
              n276 = Unbundle By Name(w168) -> ("BoardNum"=w167:u32, "SpargeBit"=w166:u32)
              n277 = call "Sparge_subVI_BM.vi"("BitNum"=w166, "BoardNum"=w167, "Sparge now"=FALSE) -> ("Sparging"=w170:bool)  [unwired: 8 in]
              n278 = local write "Sparging"(w170) -> ()
            }
            frame #6 {
              # "Wait 30 sec for sparge pressure to dissipate"
              n279 = Wait (ms)(milliseconds to wait=u32 30000) -> ()  [unwired: 1 out]
            }
            frame #7 {
              # "If run on OSSCAR, set the flow path back to the sparge chamber"
              n280 = local read "Constants"() -> (w175:T5)
              n281 = Unbundle By Name(w175) -> ("BoardNum"=w172:u32)
              n282 = Equal?(x=u32 0, y=w172) -> (x = y?=w173:bool)
              n283 = case shown="True" w173 {
                tunnel: w172 -> [_ w176]
                frame False {
                }
                frame True {
                  n284 = call "EC_switch_flow_path_subVI_BM.vi"("BoardNum"=w176, "Switch Flow Path"=FALSE) -> ()  [unwired: 10 in]
                }
              }
            }
          }
        }
      }
    }
  }
